vi "Get XYZ.vi"(8 "error in (no error)":errorcluster, 11 "VISA resource name out":refnum<visa-resource-name>) -> (0 "error out":errorcluster, 2 "XYZ":dbl[](array[numeric]), 3 "VISA resource name out 2":refnum<visa-resource-name>)   [LabVIEW 2018, in "Stage Actor.lvlib"]
uses:
  Stage Actor.lvlib
  <instrlib>/Zaber A Series/Zaber A Series.lvlib
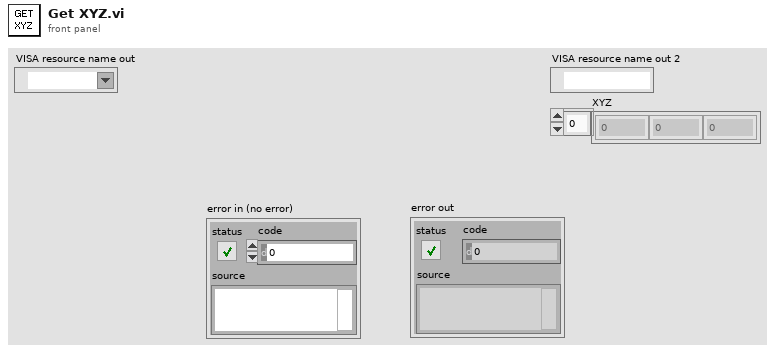
[diagram p1: front panel]
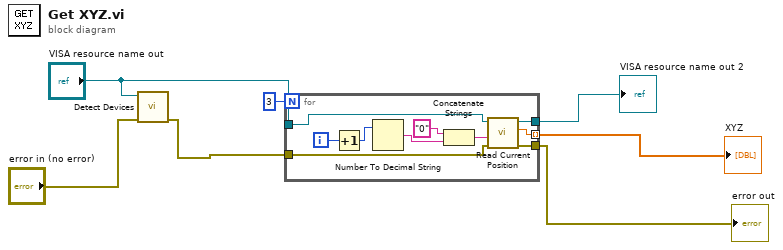
[diagram p0: block diagram]
diagram:
  n1 = call <instrlib>:"Detect Devices.vi"("error in (no error)"="error in (no error)", "VISA resource name"="VISA resource name out") -> ("error out"=w2:errorcluster)  [unwired: 6 in, 3 out]
  n2 = for {
    N: 3 -> [_]
    tunnel: "VISA resource name out" -> [w13]
    tunnel: [w12] -> w7
    tunnel: w2 -> [w11]
    tunnel: [w10] -> w6
    tunnel: [w9] -> w5 mode=indexing
    i -> [w17]
    n3 = Increment(x=w17) -> (x+1=w8:i32)
    n4 = Number To Decimal String(number=w8) -> (decimal integer string=w16:string)  [unwired: 1 in]
    n5 = Concatenate Strings("0" ("string"), w16) -> (w14:string)
    n6 = call <instrlib>:"Read Current Position.vi"("error in (no error)"=w11, "Device and Axis"=w14, "VISA resource name"=w13) -> ("error out"=w10:errorcluster, "Position"=w9:dbl, "VISA resource name out"=w12:refnum<visa-resource-name>)  [unwired: 6 in]
  }
  "VISA resource name out 2" <- w7
  "error out" <- w6
  "XYZ" <- w5
